vi "EV Rotator Initialize Editor.vi"(6 "Channel":i32=1, 8 "Calibration in":string, 9 "Hardware in":string, 10 "Setup in":string, 11 "Editor seq info":T1 {"Steps config"."Loop Info"."unit scale" items=["Log", "Lin"]; "Steps config"."Loop Info"."unit dB ref" format="%#_6p"}) -> (1 "Step name out":string="Calibration Default", 2 "Setup out":string, 3 "Sequence channels & curves out":string[](array[string]))   [LabVIEW 2018]
uses:
  custom and Sc run Seq Sub VIs (x64).llb/editor seq info.ctl
  custom and Sc run Seq Sub VIs (x64).llb/Steps config.ctl
  C:/SoundCheck 19/System/Custom VIs/EV.Rotator.RotatorControl.dll
  EV.Rotator.RotatorControl.dll
panel:
  out "Rotator Control.dll version":string
  in  "Rexroth controller IP address":string
  in  "Save as":bool
  in  "save":bool
  in  "revert":bool
  in  "continue loop?":bool
  in  "cancel":bool
  in  "load":bool
  # "This VI runs the following initialization routine:\n  - connect to Rexroth controller \n  - reset top axis encoder reference\n  - enable drives and absolute mode"
  # "Reminder:  You must edit this custom step from\nwithin a sequence for it to remember your settings."
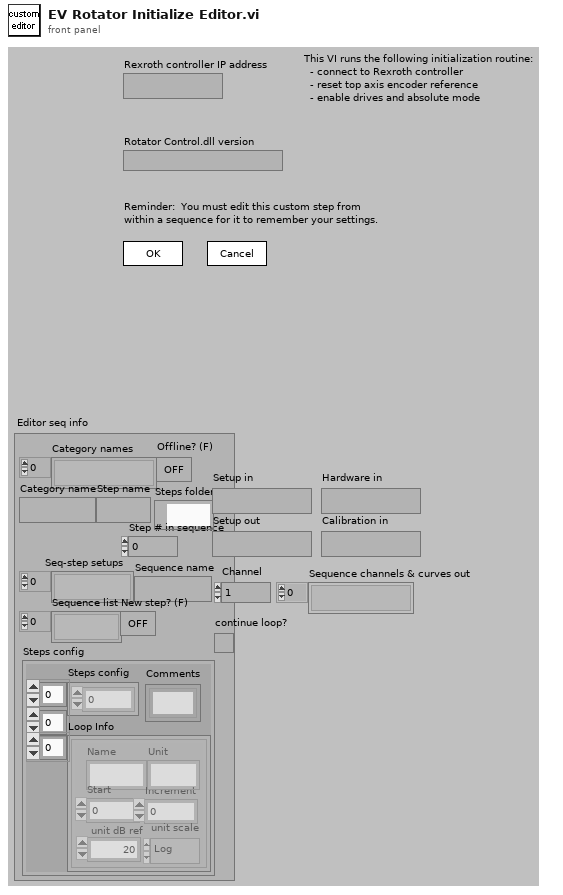
[diagram p1: front panel]
types:
  T1 = typedef "editor seq info.ctl" = cluster{"Category names":string[], "Category name":string, "Step name":string, "Step # in sequence":i32, "Seq-step setups":string[], "Sequence name":string, "Sequence list":string[], "New step? (F)":bool, "Steps config":T2, "Offline? (F)":bool, "Steps folder":path}
  T2 = typedef "Steps config.ctl" = cluster{"Steps config":i32[][], "Loop Info":cluster{"Name":string, "Start":dbl, "Increment":dbl, "Unit":string, "unit dB ref":dbl, "unit scale":u16}[], "Comments":string[]}
  T3 = cluster{"load":bool, "revert":bool, bool, "cancel":bool, "Save as":bool, bool, bool}
  T4 = cluster{"load":bool, "revert":bool, "save":bool, "cancel":bool, "Save as":bool, "close panel":bool, "apply":bool}
  T5 = typedef "seq step setup.ctl" = cluster{"Input Signal Channels":i32[], "Output Signal Channels":i32[], "Curves selected":string[][], "Curves generated":string[], "Step setup flat":string, "Trigger Signal Channel":i32, "Curves Generated Assumptions":cluster{"seq-setup in":string, "Relevant subset of mem list Grouping":cluster{T6[]}[]}}
  T6 = typedef "Memory List Grouping.ctl" = cluster{"item name":string, "parent":string, "Open?":bool, "Type":T7}
  T7 = typedef "Memory List Grouping - Item Type.ctl" = enum16{"item", "custom group", "auto group", "protected group"}
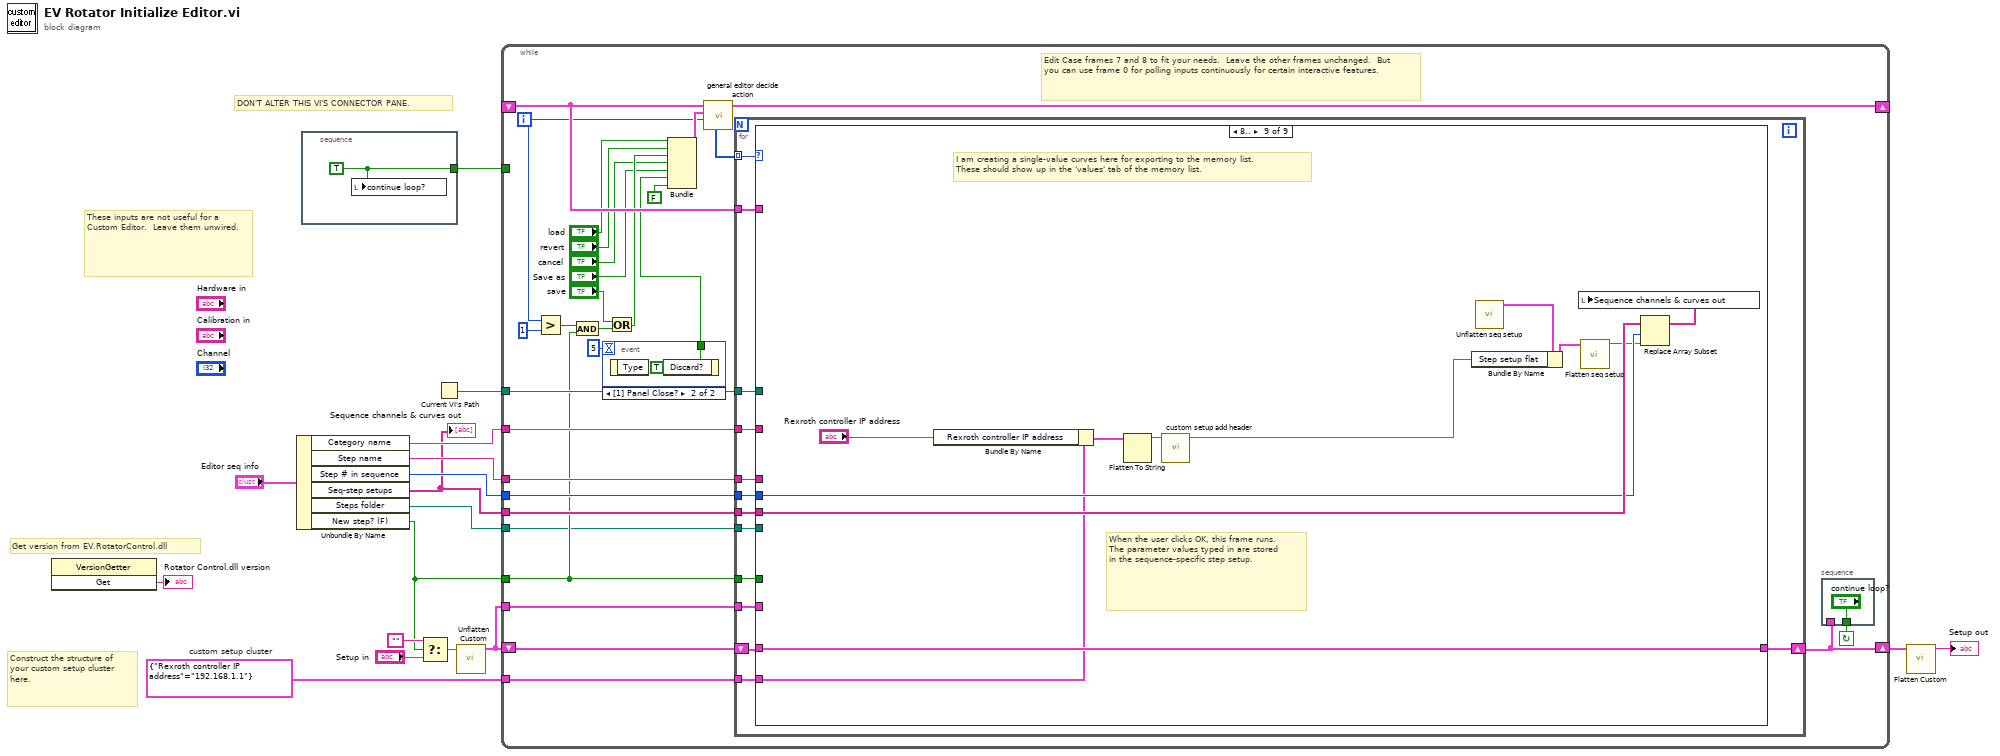
[diagram p0: block diagram]
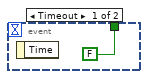
[diagram p2: hidden frame]
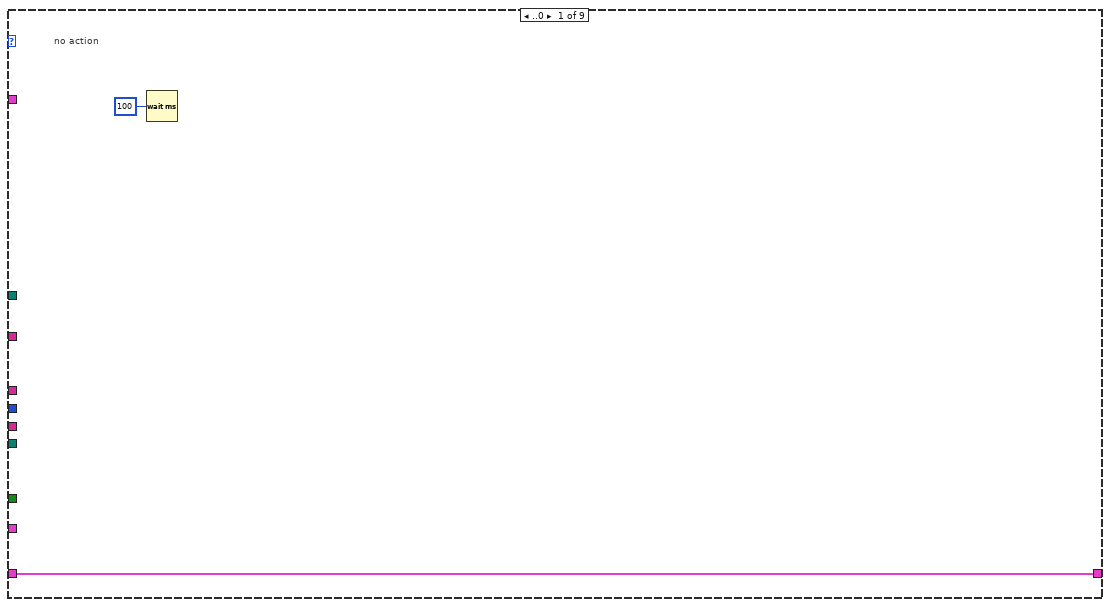
[diagram p3: hidden frame]
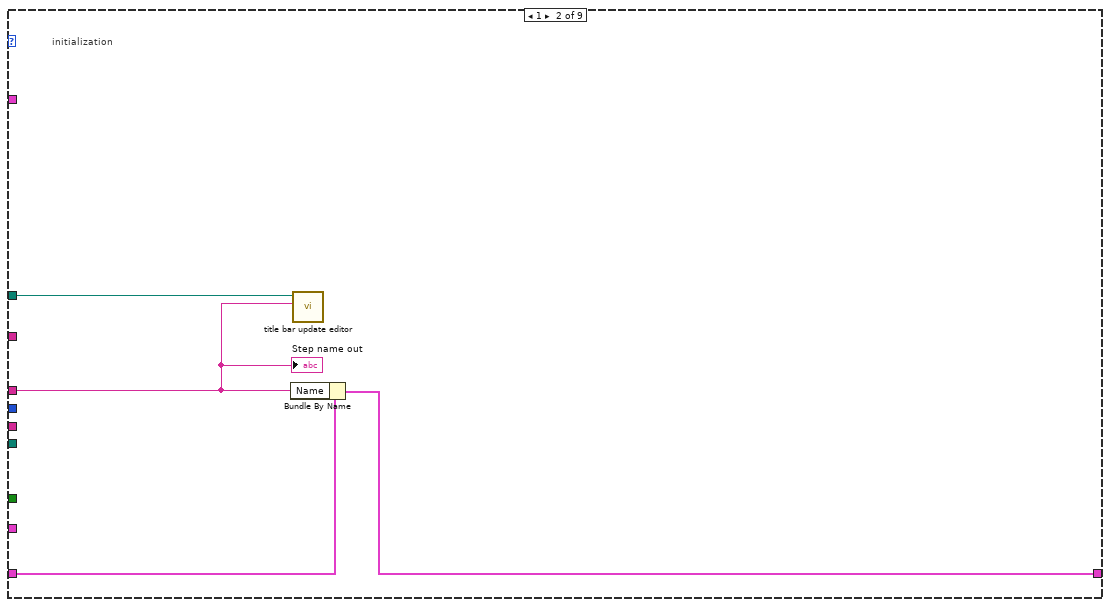
[diagram p4: hidden frame]
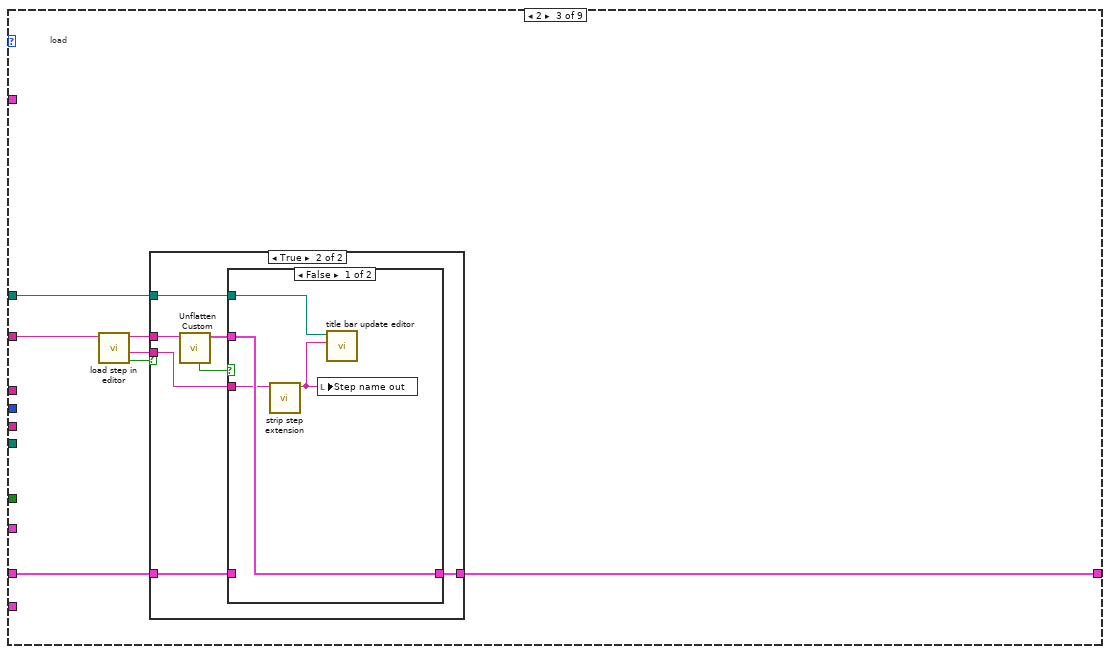
[diagram p5: hidden frame]
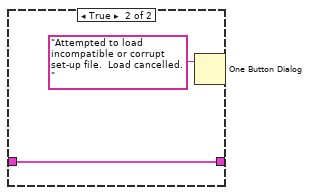
[diagram p7: hidden frame]
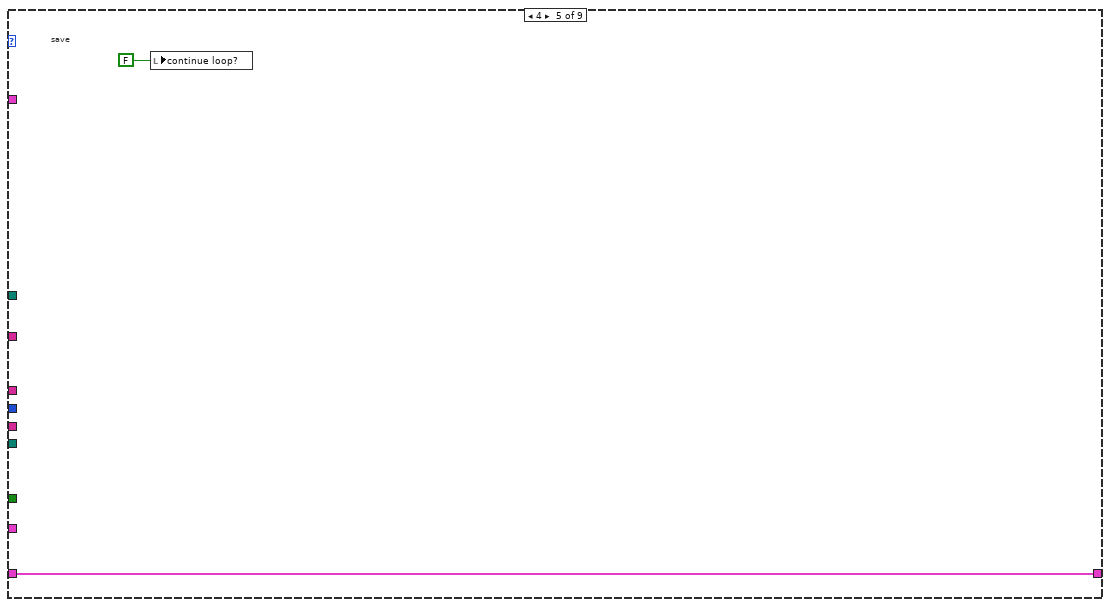
[diagram p9: hidden frame]
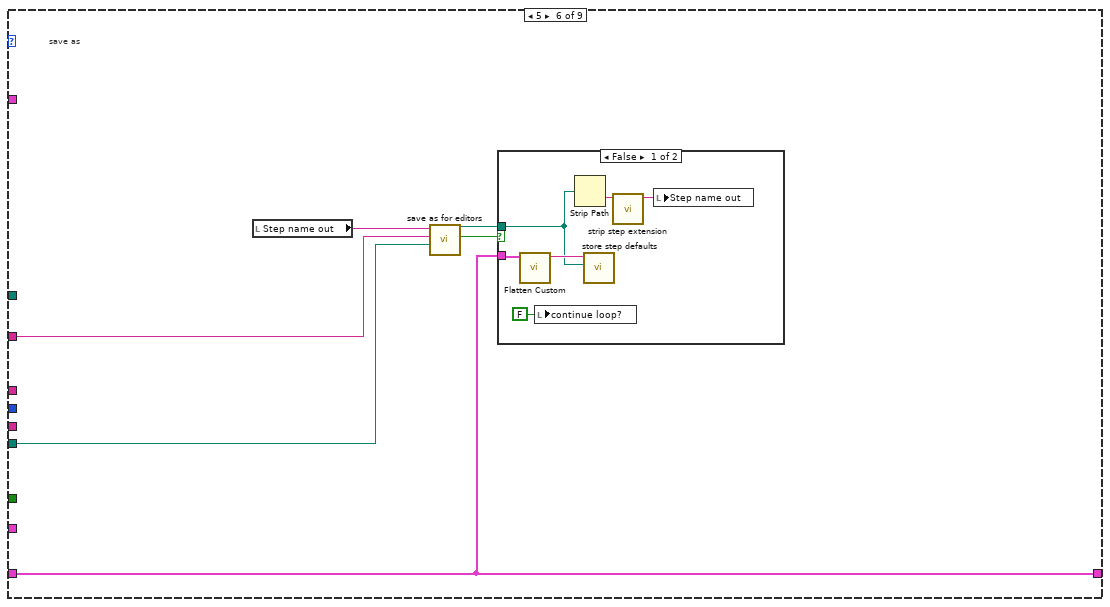
[diagram p10: hidden frame]
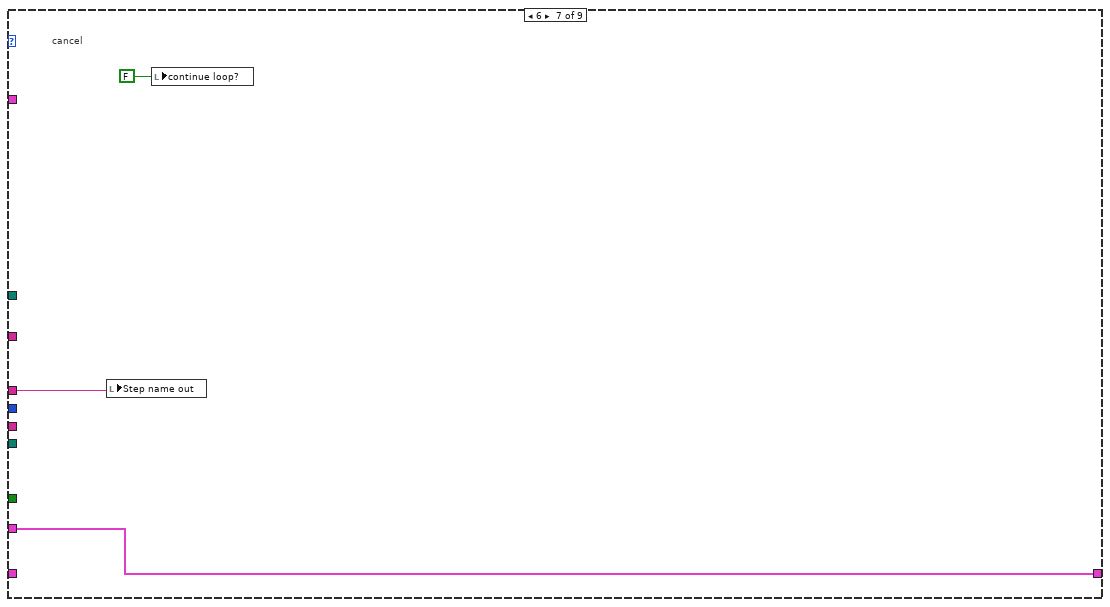
[diagram p12: hidden frame]
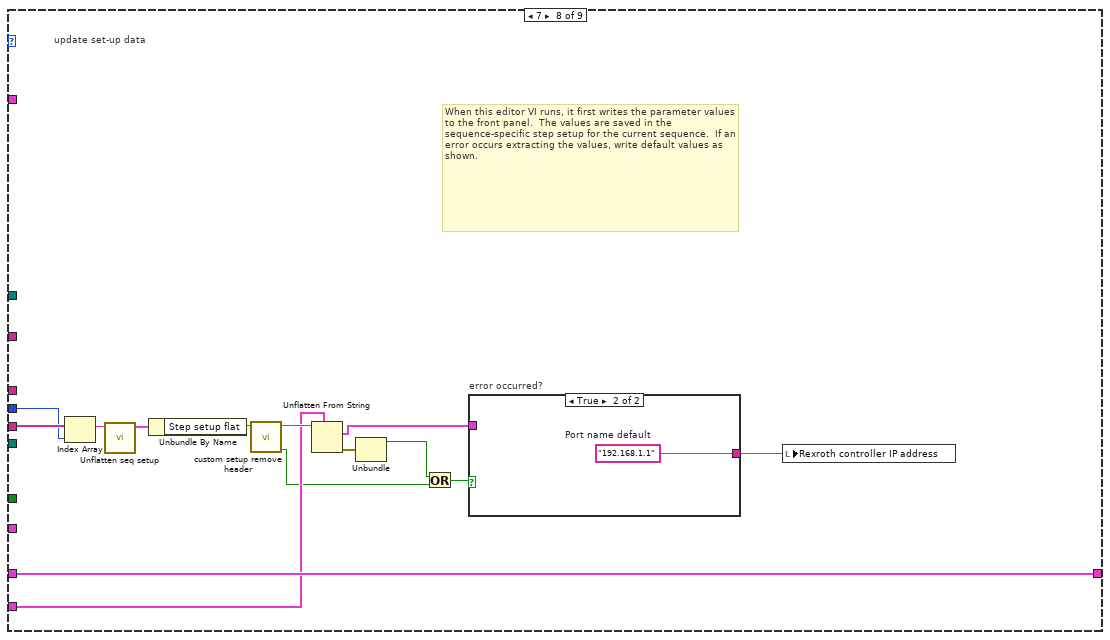
[diagram p13: hidden frame]
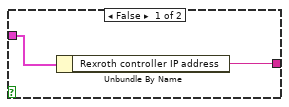
[diagram p14: hidden frame]
diagram:
  w13 = cluster{"Rexroth controller IP address":string} {"Rexroth controller IP address"="192.168.1.1"}  # custom setup cluster
  # "Get version from EV.RotatorControl.dll"
  # "Construct the structure of your custom setup cluster here."
  # "These inputs are not useful for a Custom Editor.  Leave them unwired."
  # "DON'T ALTER THIS VI'S CONNECTOR PANE."
  n1 = invoke class="VersionGetter" method="Get"() -> ("Get"=→"Rotator Control.dll version":string)  [unwired: 3 in, 2 out]
  n2 = Unbundle By Name("Editor seq info") -> ("Category name"=w10:string, "Step name"=w9:string, "Step # in sequence"=w8:i32, "Seq-step setups"=w6:string[], "Steps folder"=w7:path, "New step? (F)"=w3:bool)
  "Sequence channels & curves out" <- w6
  n3 = stacked-sequence {
    tunnel: [w18] -> w11
    frame #0 {
      w18 = TRUE ("continue loop?")
      n4 = local write "continue loop?"(w18) -> ()
    }
  }
  n5 = Select(t="", s=w3, f="Setup in") -> (s? t:f=w14:string)
  n6 = Current VI's Path() -> (path=w12:path)
  n7 = call "Unflatten Custom.vi"("Unflatten Custom"=w14) -> ("Custom"=w2:cluster{"Name":string})  [unwired: 10 out]
  n8 = while {
    tunnel: w13 -> [w28]
    tunnel: w12 -> [w36]
    shift-left: w2 -> [w38]
    shift-right: [w29] -> w4
    tunnel: w2 -> [w40]
    tunnel: w3 -> [w32]
    tunnel: w6 -> [w42]
    tunnel: w8 -> [w43]
    tunnel: w9 -> [w44]
    tunnel: w10 -> [w45]
    shift-left: _ -> [w39]
    shift-right: [w47] -> _
    tunnel: w7 -> [w25]
    tunnel: w11 -> [_]
    i -> [w35]
    stop <- w41 continue-if-true
    # "Edit Case frames 7 and 8 to fit your needs.  Leave the other frames unchanged.  But you can use frame 0 for polling inputs continuously for certain interactive features."
    n9 = Greater?(x=w35, y=1) -> (0:w33:bool)
    n10 = And(x=w33, y=w32) -> (x .and. y?=w31:bool)
    n11 = event shown="[1] Panel Close?" {
      selector: _ -> [_ _]
      dyn-events: _ -> [_ _]
      timeout: 5 -> [_ _]
      tunnel: [FALSE w49] -> w27
      event Timeout {
        n12 = event-data() -> ()  [unwired: 2 out]
      }
      event Panel Close? {
        w49 = TRUE
        n13 = event-data() -> ()  [unwired: 2 out]
        n14 = event-data("Discard?"=w49) -> ()  [unwired: 1 in, 1 out]
      }
    }
    n15 = Or(x="save", y=w31) -> (x .or. y?=w30:bool)
    n16 = Bundle("load"="load", "revert"="revert", w30, "cancel"="cancel", "Save as"="Save as", w27, FALSE) -> (w37:T3)  [unwired: 1 out]
    n17 = call "general editor decide action.vi"("Iteration"=w35, "Polled cluster"=w37, "Old cluster"=w39) -> ("actions array"=w46:i32[], "New cluster"=w47:T4)  [unwired: 1 in, 6 out]
    n18 = for {
      tunnel: w39 -> [w63]
      tunnel: w40 -> [w62]
      tunnel: w32 -> [w61]
      tunnel: w42 -> [w60]
      tunnel: w43 -> [w59]
      tunnel: w44 -> [w58]
      tunnel: w45 -> [w57]
      tunnel: w46 -> [w56] mode=indexing
      shift-right: [w54] -> w29
      shift-left: w38 -> [w55]
      tunnel: w36 -> [w53]
      tunnel: w28 -> [w52]
      tunnel: w25 -> [w51]
      n19 = case shown="8.." w56 {
        tunnel: w57 -> [_ _ w72 _ _ w96 _ _ _]
        tunnel: w58 -> [_ w66 _ _ _ _ w106 _ _]
        tunnel: w59 -> [_ _ _ _ _ _ _ w119 w134]
        tunnel: w60 -> [_ _ _ _ _ _ _ w120 w135]
        tunnel: w61 -> [_ _ _ _ _ _ _ _ _]
        tunnel: w62 -> [_ _ _ w91 _ _ w107 _ _]
        tunnel: [w64 w69 w76 w91 w92 w99 w107 w122 w131] -> w54
        tunnel: w55 -> [w64 w68 w75 _ w92 w99 _ w122 w131]
        tunnel: w63 -> [_ _ _ _ _ _ _ _ _]
        tunnel: w53 -> [_ w67 w70 _ _ _ _ _ _]
        tunnel: w52 -> [_ _ _ _ _ _ _ w115 w128]
        tunnel: w51 -> [_ _ _ _ _ w94 _ _ _]
        frame ..0 {
          # "no action"
          n20 = Wait (ms)(milliseconds to wait=u32 100) -> ()  [unwired: 1 out]
        }
        frame 1 {
          # "initialization"
          n21 = Bundle By Name(cluster=w68, "Name"=w66) -> (w69:cluster{"Name":string})
          n22 = call "title bar update editor.vi"("Step name"=w66, "Editor VI path"=w67) -> ()  [unwired: 10 out]
          "Step name out" <- w66
        }
        frame 2 {
          # "load"
          n23 = call "load step in editor.vi"("Category name"=w72) -> ("Not canceled?"=w73:bool, "New step name (with ext.)"=w71:string, "Flat step set-up"=w74:string)  [unwired: 1 in, 7 out]
          n24 = case shown="True" w73 {
            tunnel: w74 -> [_ w84]
            tunnel: [w77 w82] -> w76
            tunnel: w75 -> [w77 w81]
            tunnel: w71 -> [_ w79]
            tunnel: w70 -> [_ w78]
            frame False {
            }
            frame True {
              n25 = call "Unflatten Custom.vi"("Unflatten Custom"=w84) -> ("Custom"=w80:cluster{"Name":string}, "Error?"=w83:bool)  [unwired: 9 out]
              n26 = case shown="False" w83 {
                tunnel: [w88 w90] -> w82
                tunnel: w81 -> [_ w90]
                tunnel: w80 -> [w88 _]
                tunnel: w79 -> [w87 _]
                tunnel: w78 -> [w86 _]
                frame False {
                  n27 = call "strip step extension.vi"("Step name w/ extension"=w87) -> ("Step name (base)"=w85:string)  [unwired: 1 in, 9 out]
                  n28 = local write "Step name out"(w85) -> ()
                  n29 = call "title bar update editor.vi"("Step name"=w85, "Editor VI path"=w86) -> ()  [unwired: 10 out]
                }
                frame True {
                  n30 = One Button Dialog(message="Attempted to load incompatible or corrupt set-up file.  Load cancelled.") -> ()  [unwired: 2 out]
                }
              }
            }
          }
        }
        frame 3 {
          # "revert"
        }
        frame 4 {
          # "save"
          n31 = local write "continue loop?"(FALSE ("continue loop?")) -> ()
        }
        frame 5 {
          # "save as"
          n32 = local read "Step name out"() -> (w95:string)
          n33 = call "save as for editors.vi"("Steps Folder (gbl if empty)"=w94, "Category name"=w96, "Step name"=w95) -> ("Canceled"=w97:bool, "File path chosen"=w98:path)  [unwired: 3 in, 4 out]
          n34 = case shown="False" w97 {
            tunnel: w98 -> [w101 _]
            tunnel: w99 -> [w104 _]
            frame False {
              n35 = call "Flatten Custom.vi"("Custom"=w104) -> ("Custom flattened"=w105:string)  [unwired: 10 out]
              n36 = local write "continue loop?"(FALSE ("continue loop?")) -> ()
              n37 = Strip Path(path=w101) -> (name=w102:string)  [unwired: 1 out]
              n38 = call "store step defaults.vi"("Set-up file"=w101, "Flat step set-up"=w105) -> ()  [unwired: 4 in, 6 out]
              n39 = call "strip step extension.vi"("Step name w/ extension"=w102) -> ("Step name (base)"=w100:string)  [unwired: 1 in, 9 out]
              n40 = local write "Step name out"(w100) -> ()
            }
            frame True {
            }
          }
        }
        frame 6 {
          # "cancel"
          n41 = local write "Step name out"(w106) -> ()
          n42 = local write "continue loop?"(FALSE ("continue loop?")) -> ()
        }
        frame 7 {
          # "When this editor VI runs, it first writes the parameter values to the front panel.  The values are saved in the sequence-specific step setup for the current sequence.  If an error occurs extracting the values, write default values as shown."
          # "update set-up data"
          n43 = Index Array(array=w120, index=w119) -> (element=w121:string)
          n44 = call "Unflatten seq setup.vi"("Unflatten seq setup"=w121) -> ("Sequence-specific step set-up"=w118:T5)  [unwired: 3 in, 7 out]
          n45 = Unbundle By Name(w118) -> ("Step setup flat"=w117:string)
          n46 = call "custom setup remove header.vi"("Output from 'Step setup flat' of seq-setup structure"=w117) -> ("Error?"=w114:bool, "Flattened custom step setup cluster"=w116:string)  [unwired: 9 out]
          n47 = Unflatten From String(type=w115, binary string=w116) -> (value=w111:cluster{"Rexroth controller IP address":string}, error out=w110:errorcluster)  [unwired: 1 in, 3 out]
          n48 = Unbundle(w110) -> ("status"=w113:bool)  [unwired: 2 out]
          n49 = Or(x=w113, y=w114) -> (x .or. y?=w112:bool)
          n50 = case "error occurred?" shown="True" w112 {
            tunnel: w111 -> [w124 _]
            tunnel: [w123 w125] -> w109
            frame False {
              n51 = Unbundle By Name(w124) -> ("Rexroth controller IP address"=w123:string)
            }
            frame True {
              w125 = "192.168.1.1"  # Port name default
            }
          }
          n52 = local write "Rexroth controller IP address"(w109) -> ()
        }
        frame 8.. {
          # "I am creating a single-value curves here for exporting to the memory list.\nThese should show up in the 'values' tab of the memory list."
          # "When the user clicks OK, this frame runs.  The parameter values typed in are stored in the sequence-specific step setup."
          n53 = Bundle By Name(cluster=w128, "Rexroth controller IP address"="Rexroth controller IP address") -> (w127:cluster{"Rexroth controller IP address":string})
          n54 = Flatten To String(anything=w127) -> (data string=w129:string)  [unwired: 1 in, 4 out]
          n55 = call "custom setup add header.vi"("Flattened custom step setup cluster"=w129) -> ("Input to 'Step setup flat' of seq-setup structure"=w130:string)  [unwired: 1 in, 9 out]
          n56 = call "Unflatten seq setup.vi"() -> ("Sequence-specific step set-up"=w137:T5)  [unwired: 4 in, 7 out]
          n57 = Bundle By Name(cluster=w137, "Step setup flat"=w130) -> (w136:T5)
          n58 = call "Flatten seq setup.vi"("Sequence-specific step set-up"=w136) -> ("Seq setup flattened"=w133:string)  [unwired: 10 out]
          n59 = Replace Array Subset(array=w135, new element=w133, index=w134) -> (w132:string[])
          n60 = local write "Sequence channels & curves out"(w132) -> ()
        }
      }
    }
    n61 = stacked-sequence {
      tunnel: ["continue loop?"] -> w41
      tunnel: w29 -> [_]
      frame #0 {
      }
    }
  }
  n62 = call "Flatten Custom.vi"("Custom"=w4) -> ("Custom flattened"=→"Setup out":string)  [unwired: 10 out]
